vi "Connect.vi"(0 "reference in":refnum<class "Logger.lvclass">, 11 "error in (no error)":errorcluster) -> (4 "reference out":refnum<class "Logger.lvclass">, 15 "error out":errorcluster)   [LabVIEW 2019, in "Logger.lvclass"]
uses:
  Logger.lvclass
  Logger.lvclass/Logger.ctl
  DatabaseInterface_class/DatabaseInterface.lvclass
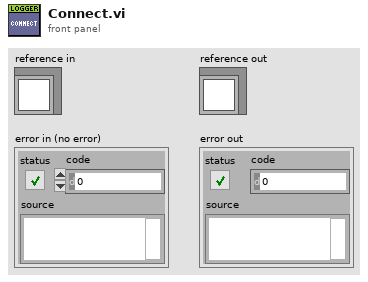
[diagram p1: front panel]
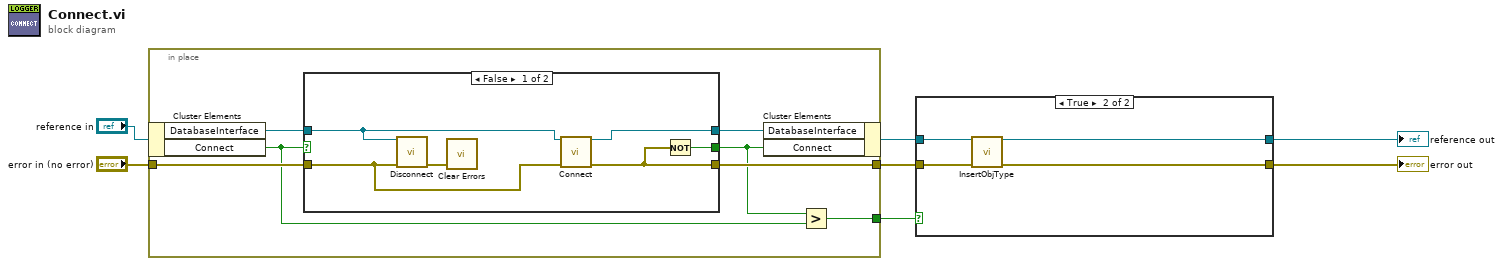
[diagram p0: block diagram]
diagram:
  n1 = in-place {
    in-place-border: "error in (no error)" -> [w13]
    in-place-border: [w12] -> w4
    in-place-border: [w8] -> w1
    n2 = in-place-cluster #1("reference in") -> ("DatabaseInterface"=w14:refnum<class "DatabaseInterface.lvclass">, "Connect"=w9:bool)
    n3 = case shown="False" w9 {
      selector: w9 -> [_ w21]
      tunnel: w14 -> [w17 w22]
      tunnel: w13 -> [w15 w23]
      tunnel: [w19 w23] -> w12
      tunnel: [w18 w22] -> w11
      tunnel: [w20 w21] -> w10
      frame False {
        n4 = call-dynamic "Disconnect.vi"("reference in"=w17, "error in (no error)"=w15) -> ("error out"=w16:errorcluster)  [unwired: 12 in, 1 out]
        n5 = call <vilib>:"Clear Errors.vi"("error in (no error)"=w16) -> ()  [unwired: 5 in, 2 out]
        n6 = call-dynamic "Connect.vi"("reference in"=w17, "error in (no error)"=w15) -> ("reference out"=w18:refnum<class "DatabaseInterface.lvclass">, "error out"=w19:errorcluster)  [unwired: 12 in]
        n7 = Not(x=w19) -> (.not. x?=w20:bool)
      }
      frame True {
      }
    }
    n8 = in-place-cluster #1("DatabaseInterface"=w11, "Connect"=w10) -> (w5:refnum<class "Logger.lvclass">)
    n9 = Greater?(x=w10, y=w9) -> (0:w8:bool)
  }
  n10 = case shown="True" w1 {
    tunnel: w5 -> [w25 w29]
    tunnel: w4 -> [w24 w28]
    tunnel: [w24 w27] -> w3
    tunnel: [w25 w26] -> w2
    frame False {
    }
    frame True {
      n11 = call "InsertObjType.vi"("reference in"=w29, "error in (no error)"=w28) -> ("reference out"=w26:refnum<class "Logger.lvclass">, "error out"=w27:errorcluster)  [unwired: 11 in, 1 out]
    }
  }
  "error out" <- w3
  "reference out" <- w2
